vi "System Explorer - Add content to System Explorer library.vi"(6 "Support Runtime Configuration":bool, 8 "error in (no error)":errorcluster, 9 "Extra Page Names":string[](array[string]), 10 "Project Root":path, 11 "CD Wizard - Internal Data":T1) -> (0 "error out":errorcluster, 1 "Extra Page VIs":path[](array[path]), 2 "System Explorer Main VI":path, 3 "Load Help File VI":path)   [LabVIEW 2020, in "NIVS_Consolidated_CDW_MetaDataObj.lvclass"]
doc: "Add all virtual folders and VIs to the System Explorer library."
uses:
  NIVS_Consolidated_CDW_MetaDataObj.lvclass
  Internal data.ctl
  CD System Explorer lvlib.ctl
  Add Item - Type.ctl
  CD System Explorer lvlib.vi
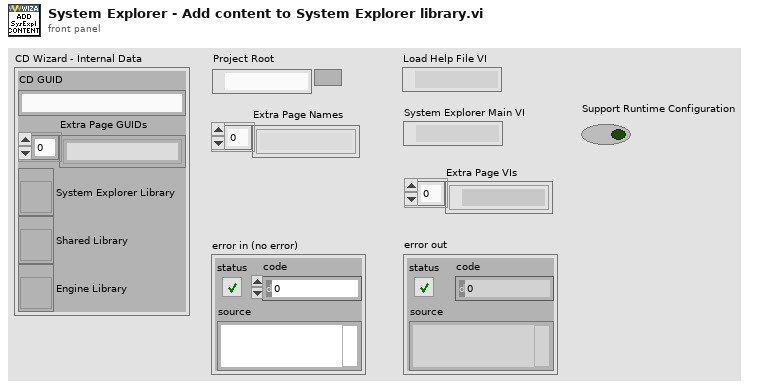
[diagram p1: front panel]
types:
  T1 = typedef "NIVS_Consolidated_CDW_MetaDataObj.lvclass/Internal data.ctl" = cluster{"CD GUID":string, "Extra Page GUIDs":string[], "System Explorer Library":refnum<vi>, "Shared Library":refnum<vi>, "Engine Library":refnum<vi>}
  T2 = typedef "NIVS_Consolidated_CDW_MetaDataObj.lvclass/CD System Explorer lvlib.ctl" = enum16{"LibraryFileName", "LibraryFolderName", "System Explorer.FolderName", "System Explorer.Dynamically Called.FolderName", "System Explorer.Dynamically Called.Extra Pages.FolderName", "System Explorer.Dynamically Called.Extra Pages.TemplatePathAndName", "System Explorer.Dynamically Called.Main Page.VIName", "System Explorer.Dynamically Called.Main Page.TemplatePathAndName", "System Explorer.Dynamically Called.Initialization VI.VIName", "System Explorer.Dynamically Called.Initialization VI.TemplatePathAndName", "System Explorer.SubVI.FolderName", "System Explorer.Types.FolderName", "System Explorer.ActionVIOnCompile.VIName", "System Explorer.ActionVIOnRecompile.VIName", "System Explorer.ExportConfigRTM.VIName", "System Explorer.PPL.ExportConfigRTM.VIName", "System Explorer.LoadHelpFile.VIName", "System Explorer.PPL.LoadHelpFile.VIName", "System Explorer.SetRTDriverVIsFilePaths.VIName", "System Explorer.ClearRTDriverVIs.VIName"}
  T3 = typedef "NIVS_Consolidated_CDW_MetaDataObj.lvclass/Add Item - Type.ctl" = string
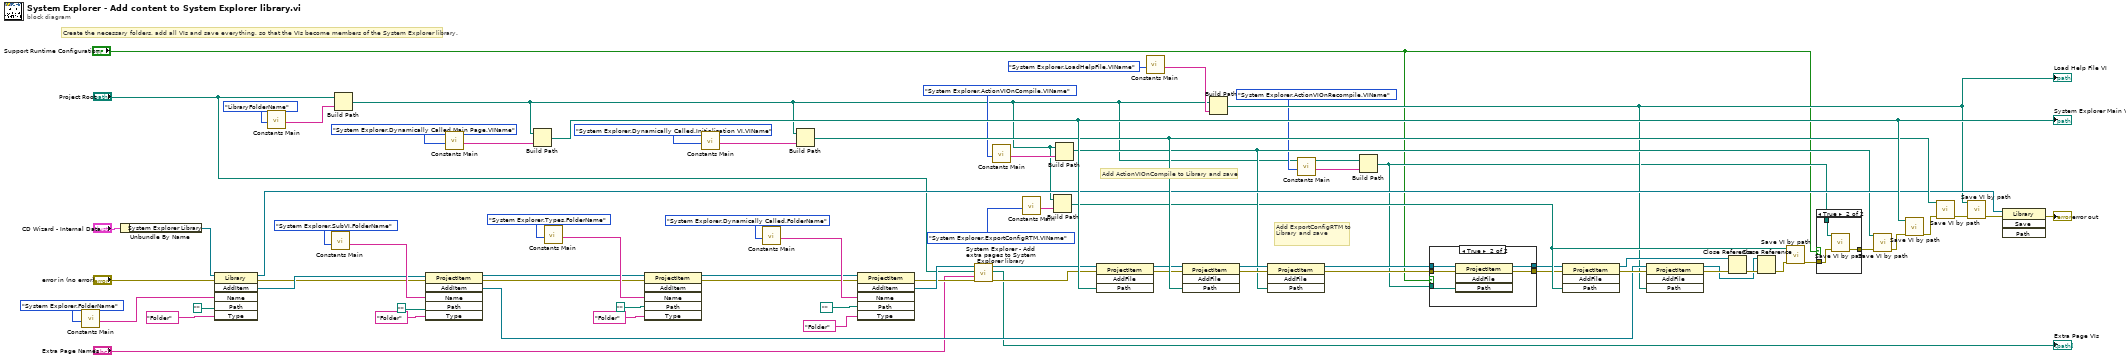
[diagram p0: block diagram]
diagram:
  # "Create the necessary folders, add all VIs and save everything, so that the VIs become members of the System Explorer library."
  # "Add ExportConfigRTM to Library and save"
  # "Add ActionVIOnCompile to Library and save"
  n1 = call-poly "Constants Main.vi"("Action"=CD_System_Explorer_lvlib."System Explorer.FolderName") -> ("Output"=w71:string)  [unwired: 10 in]
  n2 = Unbundle By Name("CD Wizard - Internal Data") -> ("System Explorer Library"=w46:refnum<vi>)
  n3 = invoke class="Library" method="AddItem"(reference=w46, error in="error in (no error)", "Name"=w71, "Path"=path "", "Type"=T3 "Folder" ("Add Item - Type")) -> (reference out=w48:refnum<vi>, error out=w19:errorcluster, "AddItem"=w47:refnum<vi>)  [unwired: 1 in, 3 out]
  n4 = call-poly "Constants Main.vi"("Action"=CD_System_Explorer_lvlib."LibraryFolderName") -> ("Output"=w41:string)  [unwired: 10 in]
  n5 = call-poly "Constants Main.vi"("Action"=CD_System_Explorer_lvlib."System Explorer.SubVI.FolderName") -> ("Output"=w63:string)  [unwired: 10 in]
  n6 = Build Path(base path="Project Root", name or relative path=w41) -> (appended path=w1:path)
  n7 = invoke class="ProjectItem" method="AddItem"(reference=w47, error in=w19, "Name"=w63, "Path"=path "", "Type"=T3 "Folder" ("Add Item - Type")) -> (reference out=w50:refnum<vi>, error out=w18:errorcluster, "AddItem"=w24:refnum<vi>)  [unwired: 1 in, 3 out]
  n8 = call-poly "Constants Main.vi"("Action"=CD_System_Explorer_lvlib."System Explorer.Dynamically Called.Main Page.VIName") -> ("Output"=w69:string)  [unwired: 10 in]
  n9 = Build Path(base path=w1, name or relative path=w69) -> (appended path=w75:path)
  "System Explorer Main VI" <- w75
  n10 = call-poly "Constants Main.vi"("Action"=CD_System_Explorer_lvlib."System Explorer.Types.FolderName") -> ("Output"=w58:string)  [unwired: 10 in]
  n11 = invoke class="ProjectItem" method="AddItem"(reference=w50, error in=w18, "Name"=w58, "Path"=path "", "Type"=T3 "Folder" ("Add Item - Type")) -> (reference out=w49:refnum<vi>, error out=w17:errorcluster)  [unwired: 1 in, 4 out]
  n12 = call-poly "Constants Main.vi"("Action"=CD_System_Explorer_lvlib."System Explorer.Dynamically Called.Initialization VI.VIName") -> ("Output"=w68:string)  [unwired: 10 in]
  n13 = call-poly "Constants Main.vi"("Action"=CD_System_Explorer_lvlib."System Explorer.Dynamically Called.FolderName") -> ("Output"=w53:string)  [unwired: 10 in]
  n14 = Build Path(base path=w1, name or relative path=w68) -> (appended path=w65:path)
  n15 = invoke class="ProjectItem" method="AddItem"(reference=w49, error in=w17, "Name"=w53, "Path"=path "", "Type"=T3 "Folder" ("Add Item - Type")) -> (error out=w43:errorcluster, "AddItem"=w45:refnum<vi>)  [unwired: 1 in, 4 out]
  n16 = call "System Explorer - Add extra pages to System Explorer library.vi"("error in (no error)"=w43, "Extra Page Names"="Extra Page Names", "Project Root"="Project Root", "ProjectItem in"=w45) -> ("error out"=w16:errorcluster, "Extra Page VIs"=→"Extra Page VIs":path[], "ProjectItem out"=w44:refnum<vi>)  [unwired: 5 in]
  n17 = call-poly "Constants Main.vi"("Action"=CD_System_Explorer_lvlib."System Explorer.ActionVIOnCompile.VIName") -> ("Output"=w35:string)  [unwired: 10 in]
  n18 = call-poly "Constants Main.vi"("Action"=CD_System_Explorer_lvlib."System Explorer.ExportConfigRTM.VIName") -> ("Output"=w31:string)  [unwired: 10 in]
  n19 = Build Path(base path=w1, name or relative path=w31) -> (appended path=w30:path)
  n20 = Build Path(base path=w1, name or relative path=w35) -> (appended path=w37:path)
  n21 = invoke class="ProjectItem" method="AddFile"(reference=w44, error in=w16, "Path"=w75) -> (reference out=w51:refnum<vi>, error out=w52:errorcluster)  [unwired: 1 in, 2 out]
  n22 = call-poly "Constants Main.vi"("Action"=CD_System_Explorer_lvlib."System Explorer.LoadHelpFile.VIName") -> ("Output"=w23:string)  [unwired: 10 in]
  n23 = invoke class="ProjectItem" method="AddFile"(reference=w51, error in=w52, "Path"=w65) -> (reference out=w40:refnum<vi>, error out=w39:errorcluster)  [unwired: 1 in, 2 out]
  n24 = Build Path(base path=w1, name or relative path=w23) -> (appended path=w11:path)
  "Load Help File VI" <- w11
  n25 = invoke class="ProjectItem" method="AddFile"(reference=w40, error in=w39, "Path"=w37) -> (reference out=w7:refnum<vi>, error out=w9:errorcluster)  [unwired: 1 in, 2 out]
  n26 = call-poly "Constants Main.vi"("Action"=CD_System_Explorer_lvlib."System Explorer.ActionVIOnRecompile.VIName") -> ("Output"=w12:string)  [unwired: 10 in]
  n27 = Build Path(base path=w1, name or relative path=w12) -> (appended path=w3:path)
  n28 = case shown="True" "Support Runtime Configuration" {
    tunnel: w9 -> [w79 w84]
    tunnel: [w79 w83] -> w8
    tunnel: w7 -> [w78 w82]
    tunnel: [w78 w81] -> w6
    tunnel: w3 -> [_ w80]
    frame False {
    }
    frame True {
      n29 = invoke class="ProjectItem" method="AddFile"(reference=w82, error in=w84, "Path"=w80) -> (reference out=w81:refnum<vi>, error out=w83:errorcluster)  [unwired: 1 in, 2 out]
    }
  }
  n30 = invoke class="ProjectItem" method="AddFile"(reference=w6, error in=w8, "Path"=w30) -> (reference out=w27:refnum<vi>, error out=w34:errorcluster)  [unwired: 1 in, 2 out]
  n31 = invoke class="ProjectItem" method="AddFile"(reference=w24, error in=w34, "Path"=w11) -> (reference out=w25:refnum<vi>, error out=w29:errorcluster)  [unwired: 1 in, 2 out]
  n32 = Close Reference(reference=w27, error in (no error)=w29) -> (error out=w33:errorcluster)
  n33 = Close Reference(reference=w25, error in (no error)=w33) -> (error out=w26:errorcluster)
  n34 = call "Save VI by path.vi"("error in (no error)"=w26, "VI path"=w30) -> ("error out"=w5:errorcluster)  [unwired: 9 in]
  n35 = case shown="True" "Support Runtime Configuration" {
    tunnel: w5 -> [w85 w88]
    tunnel: [w85 w87] -> w4
    tunnel: w3 -> [_ w86]
    frame False {
    }
    frame True {
      n36 = call "Save VI by path.vi"("error in (no error)"=w88, "VI path"=w86) -> ("error out"=w87:errorcluster)  [unwired: 9 in]
    }
  }
  n37 = call "Save VI by path.vi"("error in (no error)"=w4, "VI path"=w37) -> ("error out"=w38:errorcluster)  [unwired: 9 in]
  n38 = call "Save VI by path.vi"("error in (no error)"=w38, "VI path"=w75) -> ("error out"=w66:errorcluster)  [unwired: 9 in]
  n39 = call "Save VI by path.vi"("error in (no error)"=w66, "VI path"=w65) -> ("error out"=w22:errorcluster)  [unwired: 9 in]
  n40 = call "Save VI by path.vi"("error in (no error)"=w22, "VI path"=w11) -> ("error out"=w21:errorcluster)  [unwired: 9 in]
  n41 = invoke class="Library" method="Save"(reference=w48, error in=w21) -> (error out=→"error out":errorcluster)  [unwired: 2 in, 3 out]
